vi "Insert Value[] (String).vi"(7 "key":string[](array[string]), 8 "error in (no error)":errorcluster, 10 "JSON Data in":string, 11 "JSON Value in":refnum<class "JSON Value.lvclass">) -> (0 "error out":errorcluster, 1 "replaced":bool, 3 "JSON Value out":refnum<class "JSON Value.lvclass">)   [LabVIEW 2016, in "JSON Value.lvclass"]
uses:
  JSON Value.lvclass
  New JSON Value/New JSON (String).vi
  Insert Value (Value).vi
  Array/Replace Array Subset/Replace Array Subset (Value).vi
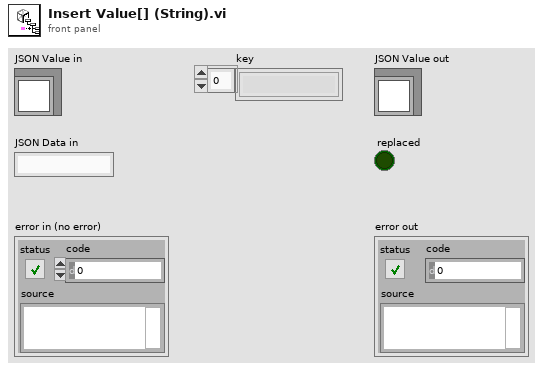
[diagram p1: front panel]
types:
  T1 = typedef "JSON Value.lvclass/JSON Types.ctl" = enum16{"String", "Numeric", "Boolean", "NULL", "Object", "Array"}
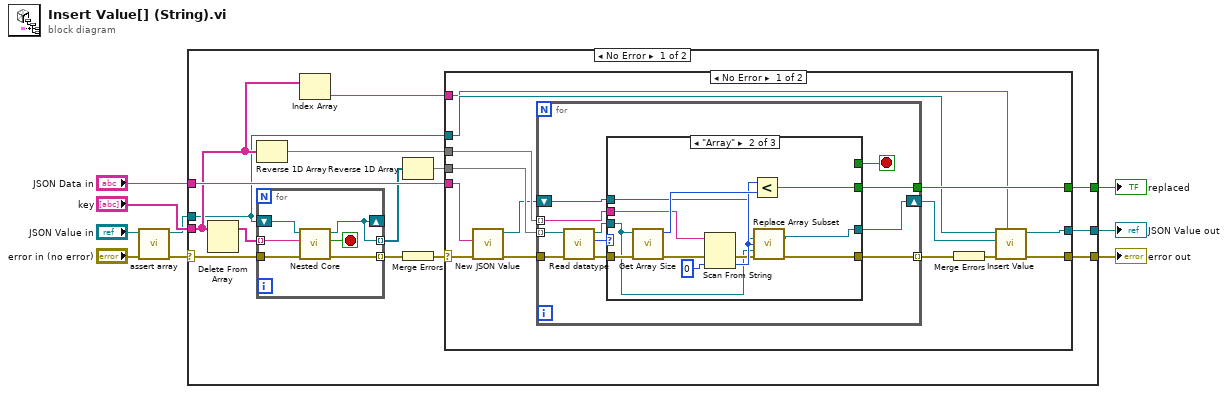
[diagram p0: block diagram]
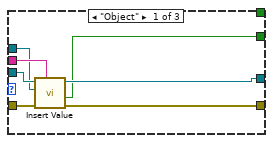
[diagram p2: hidden frame]
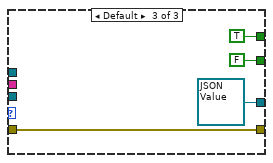
[diagram p3: hidden frame]
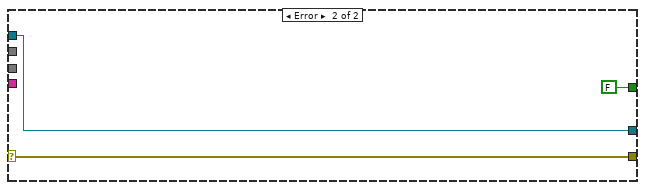
[diagram p4: hidden frame]
diagram:
  n1 = call "assert array.vi"("error in (no error)"="error in (no error)", "JSON Value in"="JSON Value in") -> ("error out"=w3:errorcluster, "JSON Value out"=w1:refnum<class "JSON Value.lvclass">)  [unwired: 8 in]
  n2 = case shown="No Error" w3 {
    selector: w3 -> [w11 w81]
    tunnel: [w23 _] -> w9
    tunnel: "JSON Data in" -> [w22 _]
    tunnel: [w15 w82] -> w6
    tunnel: [w14 w81] -> w5
    tunnel: "key" -> [w13 _]
    tunnel: w1 -> [w10 w82]
    frame No Error {
      n3 = Delete From Array(array=w13) -> (array with subset deleted=w19:string[])  [unwired: 2 in, 1 out]
      n4 = Reverse 1D Array(array=w13) -> (reversed array=w20:string[])
      n5 = for {
        tunnel: w19 -> [w80] mode=indexing
        shift-right: [w75] -> _
        shift-left: w10 -> [w79]
        tunnel: w11 -> [w78]
        tunnel: [w77] -> w16 mode=indexing
        tunnel: [w75] -> w17 mode=indexing
        stop <- w76 stop-if-true
        n6 = call "Nested Core.vi"("error in (no error)"=w78, "key"=w80, "JSON Value in"=w79) -> ("error out"=w77:errorcluster, "stop?"=w76:bool, "JSON Value out"=w75:refnum<class "JSON Value.lvclass">)  [unwired: 6 in]
      }
      n7 = Index Array(array=w13) -> (element=w12:string)  [unwired: 1 in]
      n8 = Reverse 1D Array(array=w17) -> (reversed array=w21:refnum<class "JSON Value.lvclass">[])
      n9 = Merge Errors(w16) -> (w18:errorcluster)
      n10 = case shown="No Error" w18 {
        selector: w18 -> [w25 w72]
        tunnel: [w37 FALSE ("replaced")] -> w23
        tunnel: w22 -> [w27 _]
        tunnel: w21 -> [w36 _]
        tunnel: w20 -> [w35 _]
        tunnel: [w31 w74] -> w15
        tunnel: w10 -> [w33 w74]
        tunnel: [w29 w72] -> w14
        tunnel: w12 -> [w28 _]
        frame No Error {
          n11 = call-poly "New JSON Value.vi"("error in (no error)"=w25, "value"=w27) -> ("error out"=w24:errorcluster, "JSON Value out"=w26:refnum<class "JSON Value.lvclass">)  [unwired: 8 in]
          n12 = for {
            tunnel: w35 -> [w40] mode=indexing
            tunnel: w24 -> [w46]
            tunnel: [w45] -> w34 mode=indexing
            tunnel: [w42] -> w37
            tunnel: w36 -> [w41] mode=indexing
            shift-right: [w39] -> w32
            shift-left: w26 -> [w38]
            stop <- w43 stop-if-true
            n13 = call "Read datatype.vi"("error in (no error)"=w46, "JSON Value in"=w41) -> ("error out"=w44:errorcluster, "datatype"=w47:T1, "JSON Value out"=w48:refnum<class "JSON Value.lvclass">)  [unwired: 7 in]
            n14 = case shown="\"Array\"" w47 {
              tunnel: w40 -> [w52 w64 _]
              tunnel: [w54 w56 refnum<class "JSON Value.lvclass"> refnum ("JSON Array")] -> w39
              tunnel: w48 -> [w51 w58 _]
              tunnel: [w55 w59 w70] -> w45
              tunnel: w44 -> [w50 w62 w70]
              tunnel: [_ _ TRUE] -> w43
              tunnel: [w53 w65 FALSE] -> w42
              tunnel: w38 -> [w49 w57 _]
              frame "Object" {
                n15 = call-poly "Insert Value.vi"("key"=w52, "error in (no error)"=w50, 10:"JSON Value in"=w49, 11:"JSON Value in"=w51) -> ("error out"=w55:errorcluster, "replaced"=w53:bool, "JSON Value out"=w54:refnum<class "JSON Value.lvclass">)  [unwired: 5 in]
              }
              frame "Array" {
                n16 = call "Get Array Size.vi"("error in (no error)"=w62, "JSON Value in"=w58) -> ("error out"=w61:errorcluster, "size(s)"=w66:i32)  [unwired: 8 in]
                n17 = Scan From String(input string=w64, error in=w61, default 1=0 ("index")) -> (error out=w60:errorcluster, output 1=w63:i32)  [unwired: 2 in, 2 out]
                n18 = Less?(x=w63, y=w66) -> (x < y?=w65:bool)
                n19 = call-poly "Replace Array Subset.vi"("JSON Array"=w57, "index"=w63, "new element/subarray"=w58, "error in"=w60) -> ("output JSON Array"=w56:refnum<class "JSON Value.lvclass">, "error out"=w59:errorcluster)  [unwired: 10 in]
              }
              frame Default {
              }
            }
          }
          n20 = Merge Errors(w34) -> (w30:errorcluster)
          n21 = call-poly "Insert Value.vi"("key"=w28, "error in (no error)"=w30, 10:"JSON Value in"=w32, 11:"JSON Value in"=w33) -> ("error out"=w29:errorcluster, "JSON Value out"=w31:refnum<class "JSON Value.lvclass">)  [unwired: 5 in, 1 out]
        }
        frame Error {
        }
      }
    }
    frame Error {
    }
  }
  "replaced" <- w9
  "error out" <- w5
  "JSON Value out" <- w6
